vi "Get Package File List.vi"(0 "VIPB Folder":path=path "C:/validation/Validation Framework/VI Packages/Build Specification", 5 "Package Name":string, 11 "error in (no error)":errorcluster) -> (4 "Included Files":path[](array[path]), 15 "error out":errorcluster)   [LabVIEW 2017, in "CL_G3_VIPMUtilities.lvlib"]
doc: "This VI will get list of files included in the specified package"
uses:
  CL_G3_VIPMUtilities.lvlib
  <vilib>/xml/Close Reference(Node).vi
  <vilib>/xml/Close Reference(NdList).vi
  <resource>/objmgr/DOMUserDefRef.rc
  <vilib>/xml/NI_XML.lvlib
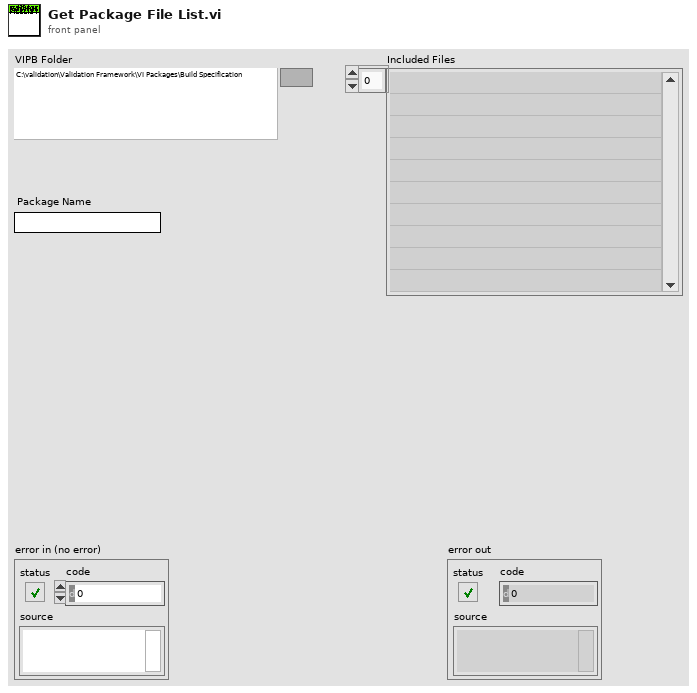
[diagram p1: front panel]
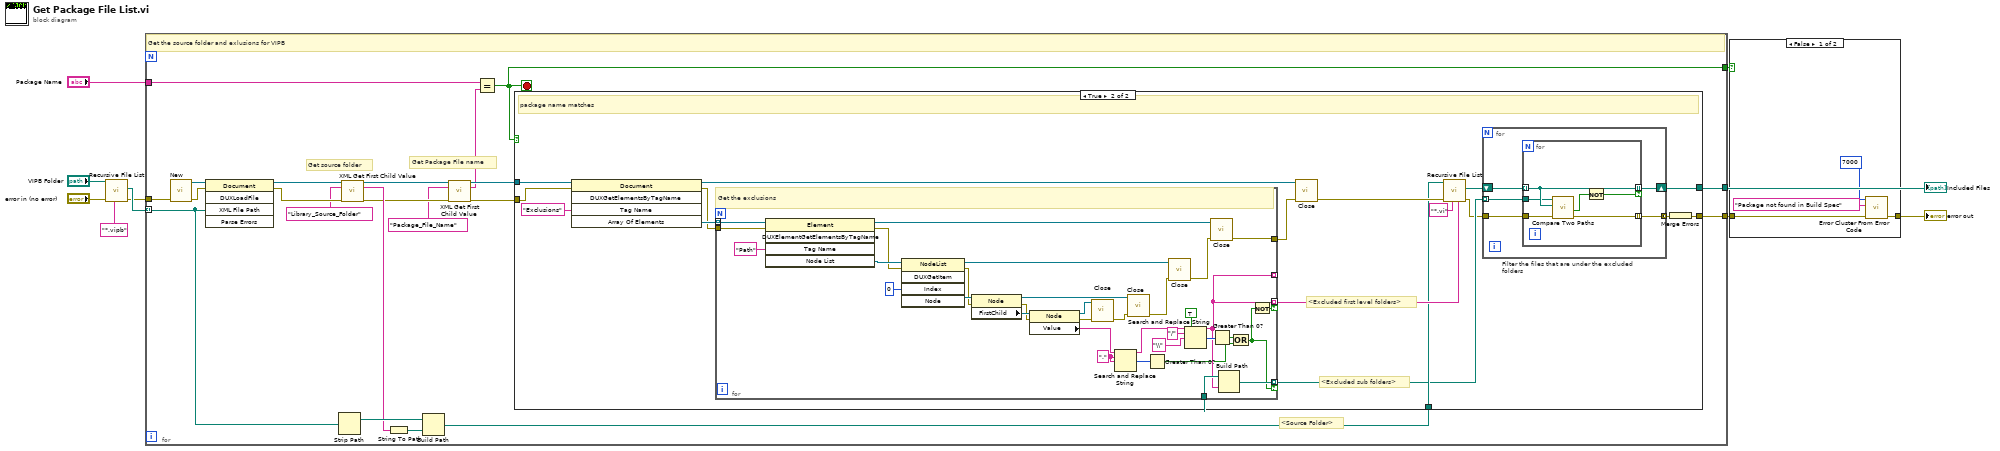
[diagram p0: block diagram]
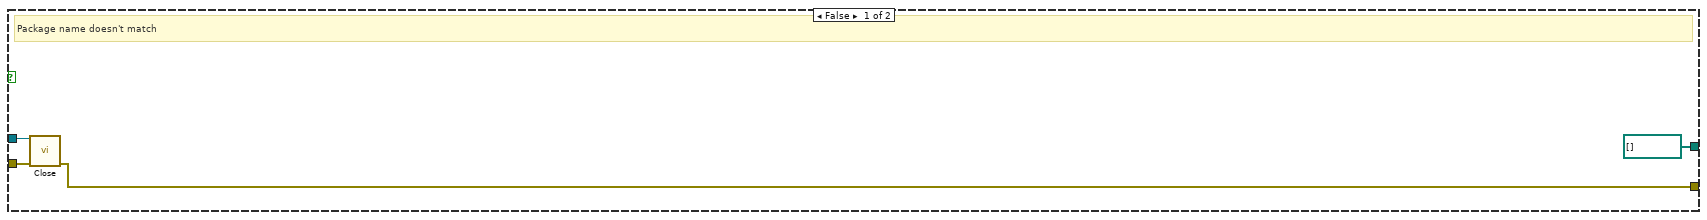
[diagram p3: hidden frame]
diagram:
  n1 = call <vilib>:"Recursive File List.vi"("pattern"="*.vipb", "error in (no error)"="error in (no error)", "Folder Path"="VIPB Folder") -> ("error out"=w4:errorcluster, "All Files in Dir"=w8:path[])  [unwired: 4 in, 3 out]
  n2 = for {
    tunnel: w4 -> [w26]
    tunnel: [w25] -> w9
    tunnel: w8 -> [w23] mode=indexing
    tunnel: [w24] -> w3
    tunnel: "Package Name" -> [w13]
    tunnel: [w11] -> w2
    stop <- w11 stop-if-true
    # "Get Package File name"
    # "Get source folder"
    # "<Source Folder>"
    # "Get the source folder and exlusions for VIPB"
    n3 = call <vilib>:"New.vi"("error in (no error)"=w26) -> ("error out"=w30:errorcluster, "DOM document out"=w31:refnum<k20>)  [unwired: 7 in]
    n4 = invoke class="Document" method="DUXLoadFile"(reference=w31, error in=w30, "XML File Path"=w23) -> (reference out=w22:refnum<k20>, error out=w21:errorcluster)  [unwired: 2 in, 3 out]
    n5 = Strip Path(path=w23) -> (stripped path=w28:path)  [unwired: 1 out]
    n6 = call "XML Get First Child Value.vi"("XML Ref In"=w22, "Tag Name"="Library_Source_Folder", "error in (no error)"=w21) -> ("XML Ref Out"=w17:refnum<k20>, "Node Value"=w19:string, "error out"=w18:errorcluster)  [unwired: 10 in]
    n7 = String To Path(string=w19) -> (path=w29:path)
    n8 = Build Path(base path=w28, name or relative path=w29) -> (appended path=w27:path)
    n9 = call "XML Get First Child Value.vi"("XML Ref In"=w17, "Tag Name"="Package_File_Name", "error in (no error)"=w18) -> ("XML Ref Out"=w15:refnum<k20>, "Node Value"=w12:string, "error out"=w16:errorcluster)  [unwired: 10 in]
    n10 = Equal?(x=w13, y=w12) -> (x = y?=w11:bool)
    n11 = case shown="True" w11 {
      tunnel: w27 -> [_ w44]
      tunnel: [path[] [] ("All Files in Dir") w40] -> w25
      tunnel: [w33 w39] -> w24
      tunnel: w16 -> [w35 w38]
      tunnel: w15 -> [w34 w37]
      frame False {
        # "Package name doesn't match"
        n12 = call-poly <vilib>:"Close.vi"("error in (no error)"=w35, "node"=w34) -> ("error out"=w33:errorcluster)  [unwired: 7 in]
      }
      frame True {
        # "<Excluded first level folders>"
        # "<Excluded sub folders>"
        # "package name matches"
        n13 = invoke class="Document" method="DUXGetElementsByTagName"(reference=w37, error in=w38, "Tag Name"="Exclusions") -> (reference out=w49:refnum<k20>, error out=w48:errorcluster, "Array Of Elements"=w51:refnum<k20>[])  [unwired: 2 in, 2 out]
        n14 = for {
          tunnel: w51 -> [w84] mode=indexing
          tunnel: [w85] -> w50
          tunnel: [w60] -> w43 mode=indexing if=w54
          tunnel: w48 -> [w75]
          tunnel: [w59] -> w46 mode=indexing if=w62
          tunnel: w44 -> [w61]
          tunnel: [w59] -> _ mode=indexing
          w56 = "." ("search string")
          # "Get the exclusions"
          n15 = invoke class="Element" method="DUXElementGetElementsByTagName"(reference=w84, error in=w75, "Tag Name"="Path") -> (reference out=w78:refnum<k20>, error out=w76:errorcluster, "Node List"=w82:refnum<k20>)  [unwired: 2 in, 2 out]
          n16 = invoke class="NodeList" method="DUXGetItem"(reference=w82, error in=w76, "Index"=0) -> (reference out=w79:refnum<k20>, error out=w74:errorcluster, "Node"=w80:refnum<k20>)  [unwired: 2 in, 2 out]
          n17 = property class="Node"(reference=w80, error in=w74) -> (reference out=w69:refnum<k20>, error out=w73:errorcluster, "FirstChild"=w77:refnum<k20>)
          n18 = property class="Node"(reference=w77, error in=w73) -> (reference out=w71:refnum<k20>, error out=w72:errorcluster, "Value"=w58:string)
          n19 = call-poly <vilib>:"Close.vi"("error in (no error)"=w72, "node"=w71) -> ("error out"=w70:errorcluster)  [unwired: 7 in]
          n20 = Search and Replace String(input string=w58, search string=w56, replace string=w56) -> (result string=w57:string, number of replacements=w55:i32)  [unwired: 5 in, 2 out]
          n21 = call-poly <vilib>:"Close.vi"("error in (no error)"=w70, "node"=w69) -> ("error out"=w68:errorcluster)  [unwired: 7 in]
          n22 = Greater Than 0?(x=w55) -> (x > 0?=w53:bool)
          n23 = call-poly <vilib>:"Close.vi"("error in (no error)"=w68, "node list"=w79) -> ("error out"=w86:errorcluster)  [unwired: 7 in]
          n24 = Search and Replace String(replace all?=TRUE ("replace all? (F)"), input string=w57, search string="/", replace string="\\" ("search string")) -> (result string=w59:string, number of replacements=w64:i32)  [unwired: 4 in, 2 out]
          n25 = call-poly <vilib>:"Close.vi"("error in (no error)"=w86, "node"=w78) -> ("error out"=w85:errorcluster)  [unwired: 7 in]
          n26 = Greater Than 0?(x=w64) -> (x > 0?=w63:bool)
          n27 = Build Path(base path=w61, name or relative path=w59) -> (appended path=w60:path)
          n28 = Or(x=w63, y=w53) -> (x .or. y?=w54:bool)
          n29 = Not(x=w54) -> (.not. x?=w62:bool)
        }
        n30 = call-poly <vilib>:"Close.vi"("error in (no error)"=w50, "node"=w49) -> ("error out"=w47:errorcluster)  [unwired: 7 in]
        n31 = call <vilib>:"Recursive File List.vi"("Folders to Exclude"=w46, "pattern"="*.vi", "error in (no error)"=w47, "Folder Path"=w44) -> ("error out"=w42:errorcluster, "All Files in Dir"=w45:path[])  [unwired: 3 in, 3 out]
        n32 = for "Filter the files that are under the excluded folders" {
          tunnel: w43 -> [w90] mode=indexing
          shift-right: [w89] -> w40
          shift-left: w45 -> [w91]
          tunnel: w42 -> [w88]
          tunnel: [w87] -> w41 mode=concatenating
          n33 = for {
            tunnel: w91 -> [w97] mode=indexing
            tunnel: [w97] -> w89 mode=indexing if=w95
            tunnel: w90 -> [w94]
            tunnel: w88 -> [w93]
            tunnel: [w92] -> w87 mode=indexing
            n34 = call <vilib>:"Compare Two Paths.vi"("error in (no error)"=w93, "Path 2"=w97, "Path 1"=w94) -> ("error out"=w92:errorcluster, "Path 2 Relative to Path 1?"=w96:bool)  [unwired: 5 in, 2 out]
            n35 = Not(x=w96) -> (.not. x?=w95:bool)
          }
        }
        n36 = Merge Errors(w41) -> (w39:errorcluster)
      }
    }
  }
  "Included Files" <- w9
  n37 = case shown="False" w2 {
    tunnel: w3 -> [w100 w102]
    tunnel: [w101 w102] -> w1
    frame False {
      n38 = call <vilib>:"Error Cluster From Error Code.vi"("error in (no error)"=w100, "error message (\"\")"="Package not found in Build Spec" ("error message (\"\")"), "error code (0)"=7000) -> ("error out"=w101:errorcluster)  [unwired: 6 in]
    }
    frame True {
    }
  }
  "error out" <- w1
